vi "TEST Create Section.vi"() -> ()   [LabVIEW 2013, in "Carya Config.lvclass"]
doc: "Copyright 2018, Carya Automatisering, Wiebe Walstra."
uses:
  Carya Config.lvclass
panel:
  out "Created session? 3":bool
  out "Session excist? 3":bool
  out "Session excist? 2":bool
  out "Session excist?":bool
  out "Created session? 2":bool
  out "Created session?":bool
  out "String 3":string
  out "String":string
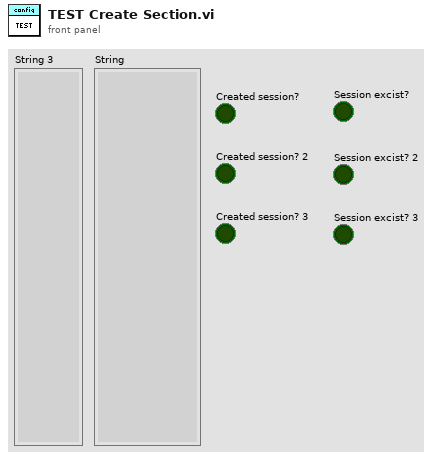
[diagram p1: front panel]
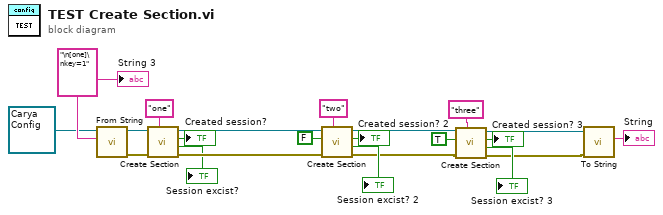
[diagram p0: block diagram]
diagram:
  w21 = "\n[one]\nkey=1" ("String")
  n1 = call-dynamic "From String.vi"("String"=w21, "Carya Config in"=refnum<class "Carya Config.lvclass"> refnum) -> ("error out"=w19:errorcluster, "Carya Config out"=w18:refnum<class "Carya Config.lvclass">)  [unwired: 7 in, 1 out]
  n2 = call-dynamic "Create Section.vi"("Section name"="one", "error in (no error)"=w19, "Carya Config in"=w18) -> ("error out"=w12:errorcluster, "Session excist?"=→"Session excist?":bool, "Created session?"=→"Created session?":bool, "Carya Config out"=w13:refnum<class "Carya Config.lvclass">)  [unwired: 5 in]
  n3 = call-dynamic "Create Section.vi"("Section name"="two", "error in (no error)"=w12, "Create section? [T]"=FALSE, "Carya Config in"=w13) -> ("error out"=w3:errorcluster, "Session excist?"=→"Session excist? 2":bool, "Created session?"=→"Created session? 2":bool, "Carya Config out"=w4:refnum<class "Carya Config.lvclass">)  [unwired: 4 in]
  n4 = call-dynamic "Create Section.vi"("Section name"="three", "error in (no error)"=w3, "Create section? [T]"=TRUE, "Carya Config in"=w4) -> ("error out"=w2:errorcluster, "Session excist?"=→"Session excist? 3":bool, "Created session?"=→"Created session? 3":bool, "Carya Config out"=w1:refnum<class "Carya Config.lvclass">)  [unwired: 4 in]
  n5 = call-dynamic "To String.vi"("error in (no error)"=w2, "Carya Config in"=w1) -> ("String"=→"String":string)  [unwired: 7 in, 2 out]
  "String 3" <- w21
